vi "DSClose.vi"(8 "error in (no error)":errorcluster[](array[cluster]), 11 "connection id":refnum<k13>[](array[refnum])) -> ()   [LabVIEW 2011]
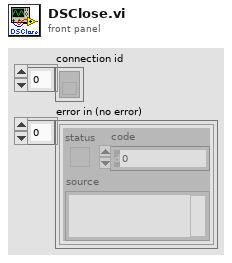
[diagram p1: front panel]
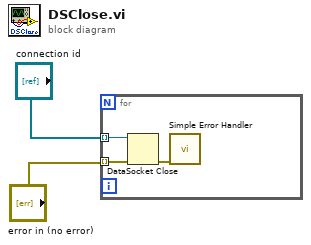
[diagram p0: block diagram]
diagram:
  n1 = for {
    tunnel: "connection id" -> [w5] mode=indexing
    tunnel: "error in (no error)" -> [w3] mode=indexing
    n2 = DataSocket Close(8:w3, 11:w5) -> (0:w4:errorcluster)  [unwired: 2 out]
    n3 = call <vilib>:"Simple Error Handler.vi"("error in (no error)"=w4) -> ()  [unwired: 4 in, 5 out]
  }
